vi "Receive.vi"(11 "Dev Actor in":refnum<class "Dev Actor.lvclass">) -> (2 "Msg":refnum<class "Msg.lvclass">, 3 "Dev Actor out":refnum<class "Dev Actor.lvclass">)   [LabVIEW 2021, in "Dev Actor.lvlib" / "Dev Actor.lvclass"]
uses:
  Dev Actor.lvclass
  src/Actor/Msg/Msg.lvclass
  Dev Actor.lvclass/Dev Actor.ctl
  src/Actor/Actor/Actor.lvclass
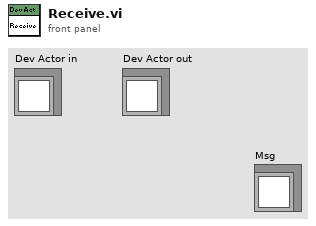
[diagram p1: front panel]
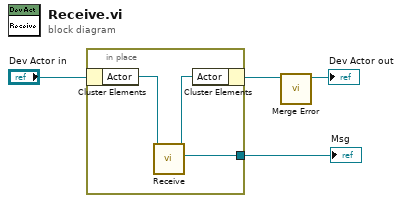
[diagram p0: block diagram]
diagram:
  n1 = in-place {
    in-place-border: [w7] -> w3
    n2 = in-place-cluster #1("Dev Actor in") -> ("Actor"=w5:refnum<class "Actor.lvclass">)
    n3 = call-dynamic "Receive.vi"("Actor in"=w5) -> ("Msg"=w7:refnum<class "Msg.lvclass">, "Actor out"=w6:refnum<class "Actor.lvclass">)  [unwired: 9 in]
    n4 = in-place-cluster #1("Actor"=w6) -> (w2:refnum<class "Dev Actor.lvclass">)
  }
  "Msg" <- w3
  n5 = call-dynamic "Merge Error.vi"("Dev Actor in"=w2) -> ("Dev Actor out"=→"Dev Actor out":refnum<class "Dev Actor.lvclass">)  [unwired: 10 in]
